vi "Local Configuration.LAS1BA.Local Base Address.Get.vi"(8 "error in (no error)":errorcluster, 11 "GE 5565PIORC":refnum<class "GE 5565PIORC Old.lvclass">) -> (0 "error out":errorcluster, 2 "Local Base Address":u32 format="%.0x", 3 "GE 5565PIORC out":refnum<class "GE 5565PIORC Old.lvclass">)   [LabVIEW 2016, in "GE 5565PIORC Old.lvclass"]
uses:
  GE 5565PIORC Old.lvclass
  <vilib>/Instr/_visa.llb/VISA Register Access Address Space.ctl
  Controls/Registers.Local Configuration.ctl
  GE 5565PIORC Old.lvclass/GE 5565PIORC Old.ctl
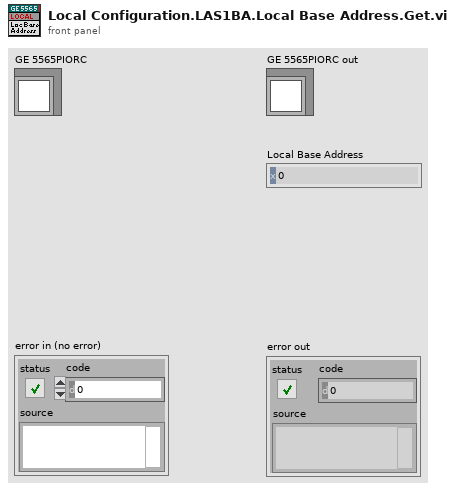
[diagram p1: front panel]
types:
  T1 = typedef "GE 5565PIORC Old.lvclass/Registers.Local Configuration.ctl" = enum16{"DMA Arbitration", "Interrupt Control and Status", "DMA Mode", "DMA PCI Address", "DMA Local Address", "DMA Transfer Size", "DMA Descriptor Pointer", "DMA Command/Status", "DMA PCI DAC Upper Address", "PCI PIO Address Range", "PCI PIO Base Address (Remap)"}
  T2 = typedef "VISA Register Access Address Space.ctl" = u16
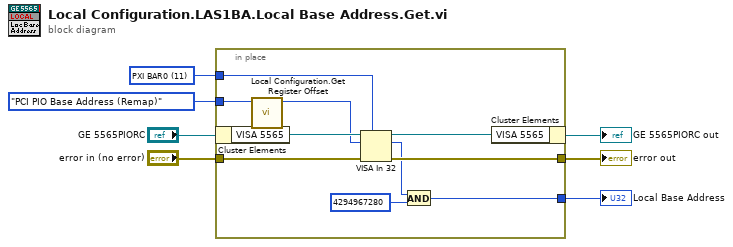
[diagram p0: block diagram]
diagram:
  w3 = T2 11 items=["VXI/VME A16"=1, "VXI/VME A24"=2, "VXI/VME A32"=3, "VXI/VME A64"=4, "PXI Memory Allocations"=9, "PXI Configuration"=10, "PXI BAR0"=11, "PXI BAR1"=12, "PXI BAR2"=13, "PXI BAR3"=14, "PXI BAR4"=15, "PXI BAR5"=16] ("Address Space")
  n1 = in-place {
    in-place-border: "error in (no error)" -> [w15]
    in-place-border: [w14] -> w5
    in-place-border: w3 -> [w12]
    in-place-border: Registers.Local_Configuration."PCI PIO Base Address (Remap)" ("Local Configration Register Offset") -> [w11]
    in-place-border: [w8] -> w1
    n2 = in-place-cluster #1("GE 5565PIORC") -> ("VISA 5565"=w17:refnum<visa-resource-name>)
    n3 = call "Local Configuration.Get Register Offset.vi"("Local Configuration Register"=w11) -> ("Offset"=w13:u32)  [unwired: 10 in]
    n4 = VISA In 32(7:w12, 8:w15, 10:w13, 11:w17) -> (0:w14:errorcluster, 2:w9:u32, 3:w16:refnum<visa-resource-name>)
    n5 = And(x=w9, y=u32 4294967280 ("value")) -> (x .and. y?=w8:u32)
    n6 = in-place-cluster #1("VISA 5565"=w16) -> (→"GE 5565PIORC out":refnum<class "GE 5565PIORC Old.lvclass">)
  }
  "error out" <- w5
  "Local Base Address" <- w1
